vi "Register.vi"(8 "error in":errorcluster, 10 "gRPC ID in":T1, 11 "measurement service v2 in":refnum<class "Measurement Service V2.lvclass">) -> (0 "error out":errorcluster, 2 "gRPC ID out":T1, 3 "measurement service v2 out":refnum<class "Measurement Service V2.lvclass">)   [LabVIEW 2021, in "NI Measurement Plug-In SDK.lvlib" / "Measurement Service V2.lvclass"]
uses:
  Measurement Service V2.lvclass
  <vilib>/gRPC/LabVIEW gRPC Library/Shared/grpcId.ctl
  Measurement Service V2.lvclass/Measurement Service V2.ctl
  gRPC/Generated APIs/ni/measurementlink/measurement/v2/RPC Service/MeasurementService/MeasurementServiceBaseV2.lvclass/MeasurementServiceBaseV2.ctl
  gRPC/Generated APIs/ni/measurementlink/measurement/v2/RPC Service/MeasurementService/Accessor/Read Server RPC Methods.vi
  gRPC/Generated APIs/ni/measurementlink/measurement/v2/RPC Service/MeasurementService/MeasurementServiceBaseV2.lvclass
  C:/Program Files/National Instruments/LabVIEW 2024/vi.lib/gRPC/LabVIEW gRPC Servicer/ServiceBase/ServiceBase.lvclass
  gRPC/Generated APIs/ni/measurementlink/measurement/v2/ni.measurementlink.measurement.v2.api.lvlib
  <vilib>/gRPC/LabVIEW gRPC Library/grpc-lvsupport-release.lvlib
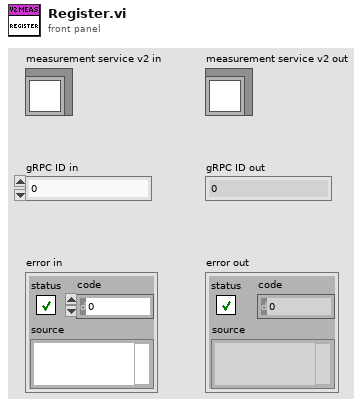
[diagram p1: front panel]
types:
  T1 = typedef "grpc-lvsupport-release.lvlib/grpcId.ctl" = u64
  T2 = typedef "ni.measurementlink.measurement.v2.api.lvlib/MeasurementServiceBaseV2.lvclass/Server gRPC UEs.ctl" = cluster{"MeasurementService GetMetadata gRPC UE":refnum<user-event>, "MeasurementService Measure gRPC UE":refnum<user-event>}
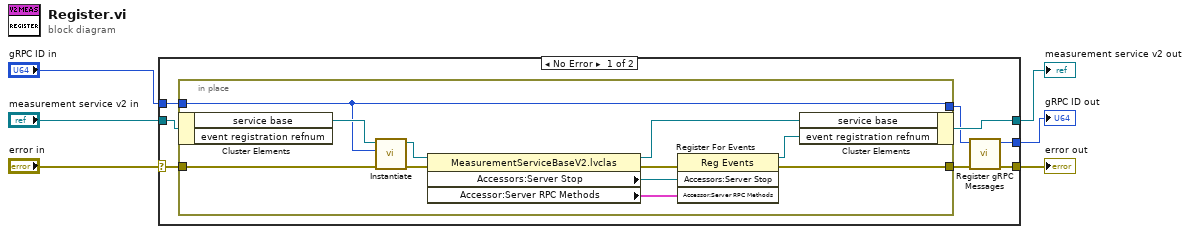
[diagram p0: block diagram]
diagram:
  n1 = case shown="No Error" "error in" {
    selector: "error in" -> [w9 w28]
    tunnel: [w13 w28] -> w5
    tunnel: [w10 w27] -> w3
    tunnel: "measurement service v2 in" -> [w11 w27]
    tunnel: "gRPC ID in" -> [w8 w26]
    tunnel: [w14 w26] -> w1
    frame No Error {
      n2 = in-place {
        in-place-border: [w17] -> w12
        in-place-border: w9 -> [w24]
        in-place-border: w8 -> [w23]
        in-place-border: [w23] -> w7
        n3 = in-place-cluster #1(w11) -> ("service base"=w25:refnum<class "MeasurementServiceBaseV2.lvclass">)  [unwired: 1 out]
        n4 = call-dynamic "Instantiate.vi"("error in"=w24, "gRPCid"=w23, "iService"=w25) -> ("error out"=w18:errorcluster, "iService"=w16:refnum<class "MeasurementServiceBaseV2.lvclass">)  [unwired: 7 in]
        n5 = property class="MeasurementServiceBaseV2.lvclas"(reference=w16, error in=w18) -> (reference out=w15:refnum<class "MeasurementServiceBaseV2.lvclass">, error out=w21:errorcluster, "Accessors:Server Stop"=w22:refnum<user-event>, "Accessor:Server RPC Methods"=w20:T2)
        n6 = register-events(error in=w21, w22, w20) -> (reference out=w19:refnum<event-registration>, error out=w17:errorcluster)  [unwired: 1 in]
        n7 = in-place-cluster #1("service base"=w15, "event registration refnum"=w19) -> (w10:refnum<class "Measurement Service V2.lvclass">)
      }
      n8 = call "Register gRPC Messages.vi"("error in (no error)"=w12, "gRPC ID"=w7) -> ("error out"=w13:errorcluster, "gRPC ID Out"=w14:T1)  [unwired: 8 in]
    }
    frame Error {
    }
  }
  "error out" <- w5
  "measurement service v2 out" <- w3
  "gRPC ID out" <- w1
